vi "trigonom.vi"() -> ()   [LabVIEW 2021]
panel:
  in  "enter B":dbl
  in  "enter phi2":dbl
  in  "enter omega2 2":dbl
  out "Plot is":string
  in  "enter A":dbl
  in  "enter omega1":dbl
  in  "enter phi1":dbl
  in  "Enum":T1(ring)
  out "cosinusoida":dbl[](graph)
  # "your omega must be in range 0-200"
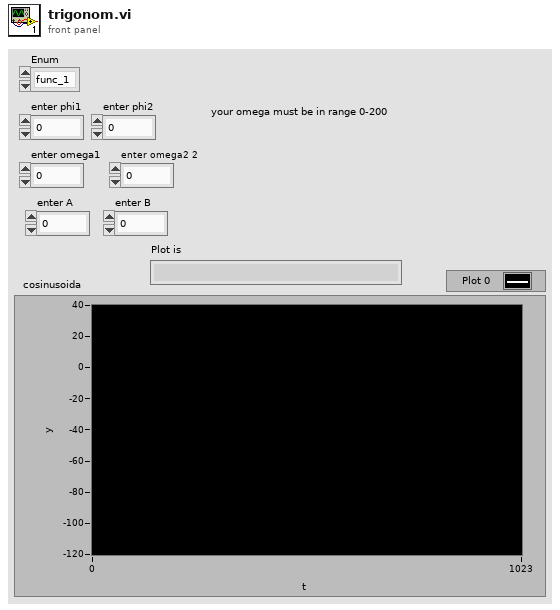
[diagram p1: front panel]
types:
  T1 = enum16{"func_1", "func_2", "func_3", "func_4", "func_5", "func_6"}
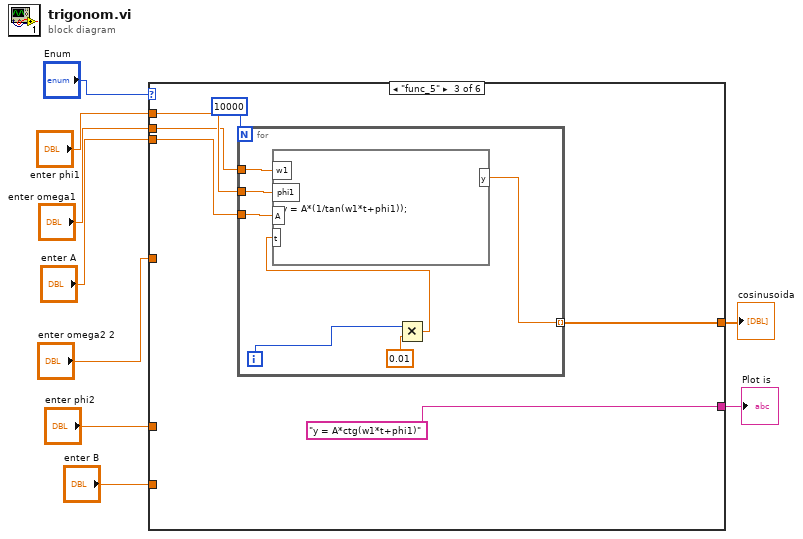
[diagram p0: block diagram]
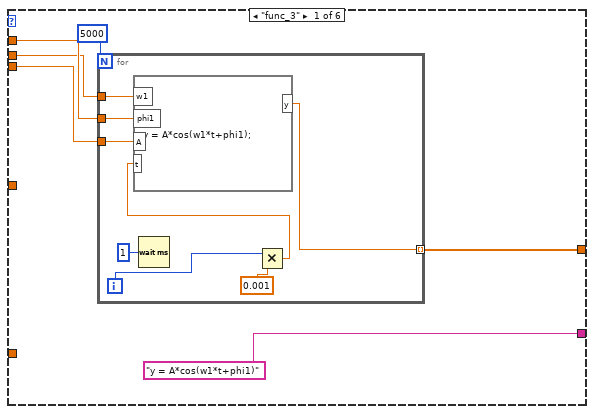
[diagram p2: hidden frame]
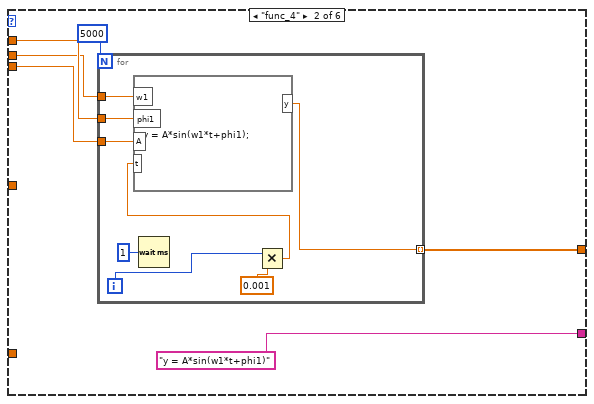
[diagram p3: hidden frame]
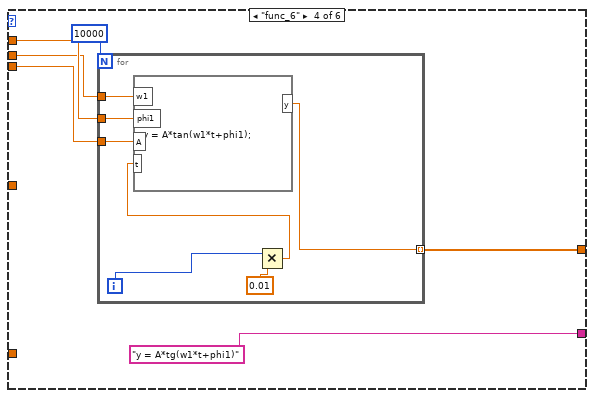
[diagram p4: hidden frame]
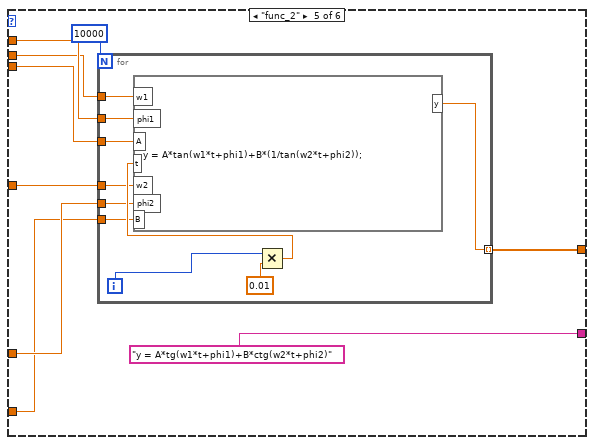
[diagram p5: hidden frame]
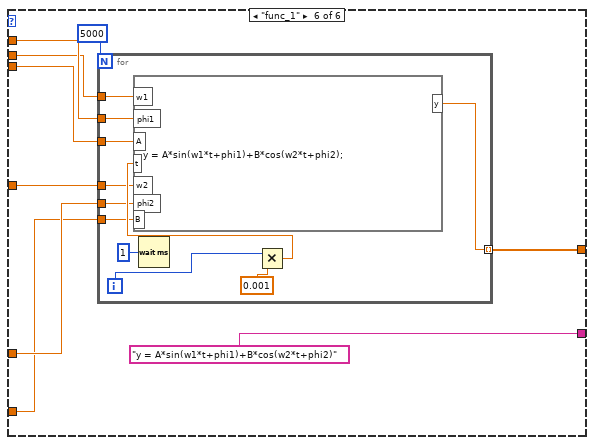
[diagram p6: hidden frame]
diagram:
  n1 = case shown="\"func_5\"" "Enum" {
    tunnel: "enter phi1" -> [w15 w29 w43 w56 w72 w91]
    tunnel: "enter omega1" -> [w14 w28 w42 w55 w71 w90]
    tunnel: "enter A" -> [w13 w27 w41 w54 w70 w89]
    tunnel: [w11 w25 w39 w52 w68 w87] -> w5
    tunnel: ["y = A*cos(w1*t+phi1)" "y = A*sin(w1*t+phi1)" "y = A*ctg(w1*t+phi1)" "y = A*tg(w1*t+phi1)" "y = A*tg(w1*t+phi1)+B*ctg(w2*t+phi2)" "y = A*sin(w1*t+phi1)+B*cos(w2*t+phi2)"] -> w4
    tunnel: "enter omega2 2" -> [_ _ _ _ w66 w85]
    tunnel: "enter phi2" -> [_ _ _ _ w65 w84]
    tunnel: "enter B" -> [_ _ _ _ w64 w83]
    frame "func_3" {
      n2 = for {
        N: 5000 -> [_]
        tunnel: w15 -> [w23]
        tunnel: w14 -> [w22]
        tunnel: w13 -> [w21]
        tunnel: [w19] -> w11 mode=indexing
        i -> [w18]
        n3 = Wait (ms)(milliseconds to wait=u32 1) -> ()  [unwired: 1 out]
        n4 = Multiply(x=w18, y=0.001) -> (x*y=w16:dbl)
        n5 = formula code="y = A*cos(w1*t+phi1);"("phi1"=w23, "w1"=w22, "A"=w21, "t"=w16) -> ("y"=w19:dbl)
      }
    }
    frame "func_4" {
      n6 = for {
        N: 5000 -> [_]
        tunnel: w29 -> [w37]
        tunnel: w28 -> [w36]
        tunnel: w27 -> [w35]
        tunnel: [w33] -> w25 mode=indexing
        i -> [w32]
        n7 = Wait (ms)(milliseconds to wait=u32 1) -> ()  [unwired: 1 out]
        n8 = Multiply(x=w32, y=0.001) -> (x*y=w30:dbl)
        n9 = formula code="y = A*sin(w1*t+phi1);"("phi1"=w37, "w1"=w36, "A"=w35, "t"=w30) -> ("y"=w33:dbl)
      }
    }
    frame "func_5" {
      n10 = for {
        N: 10000 -> [_]
        tunnel: w43 -> [w50]
        tunnel: w42 -> [w49]
        tunnel: w41 -> [w48]
        tunnel: [w47] -> w39 mode=indexing
        i -> [w46]
        n11 = Multiply(x=w46, y=0.01) -> (x*y=w44:dbl)
        n12 = formula code="y = A*(1/tan(w1*t+phi1));"("phi1"=w50, "w1"=w49, "A"=w48, "t"=w44) -> ("y"=w47:dbl)
      }
    }
    frame "func_6" {
      n13 = for {
        N: 10000 -> [_]
        tunnel: w56 -> [w63]
        tunnel: w55 -> [w62]
        tunnel: w54 -> [w61]
        tunnel: [w60] -> w52 mode=indexing
        i -> [w59]
        n14 = Multiply(x=w59, y=0.01) -> (x*y=w57:dbl)
        n15 = formula code="y = A*tan(w1*t+phi1);"("phi1"=w63, "w1"=w62, "A"=w61, "t"=w57) -> ("y"=w60:dbl)
      }
    }
    frame "func_2" {
      n16 = for {
        N: 10000 -> [_]
        tunnel: w72 -> [w82]
        tunnel: w71 -> [w81]
        tunnel: w70 -> [w80]
        tunnel: [w79] -> w68 mode=indexing
        tunnel: w66 -> [w75]
        tunnel: w65 -> [w74]
        tunnel: w64 -> [w73]
        i -> [w78]
        n17 = Multiply(x=w78, y=0.01) -> (x*y=w76:dbl)
        n18 = formula code="y = A*tan(w1*t+phi1)+B*(1/tan(w2*t+phi2));"("phi1"=w82, "w1"=w81, "A"=w80, "t"=w76, "w2"=w75, "phi2"=w74, "B"=w73) -> ("y"=w79:dbl)
      }
    }
    frame "func_1" {
      n19 = for {
        N: 5000 -> [_]
        tunnel: w91 -> [w102]
        tunnel: w90 -> [w101]
        tunnel: w89 -> [w100]
        tunnel: [w98] -> w87 mode=indexing
        tunnel: w85 -> [w94]
        tunnel: w84 -> [w93]
        tunnel: w83 -> [w92]
        i -> [w97]
        n20 = Wait (ms)(milliseconds to wait=u32 1) -> ()  [unwired: 1 out]
        n21 = Multiply(x=w97, y=0.001) -> (x*y=w95:dbl)
        n22 = formula code="y = A*sin(w1*t+phi1)+B*cos(w2*t+phi2);"("phi1"=w102, "w1"=w101, "A"=w100, "t"=w95, "w2"=w94, "phi2"=w93, "B"=w92) -> ("y"=w98:dbl)
      }
    }
  }
  "cosinusoida" <- w5
  "Plot is" <- w4
